vi "Select Worksheet for Logging.vi"(11 "Excel Logger.lvclass":refnum<class "Excel Logger.lvclass">) -> (0 "Canceled":bool=TRUE, 3 "Excel Logger.lvclass 2":refnum<class "Excel Logger.lvclass">)   [LabVIEW 2013, in "Excel Logger.lvclass"]
uses:
  Excel Logger.lvclass
  Excel Logger.lvclass/Excel Logger.ctl
  Excel Interface/Excel Interface.lvclass
  Data Analyser Report/Data Analyser Report.lvclass
panel:
  in  "Text":bool
  in  "Cancel":bool
  in  "OK Button":bool
  # "Please sellect now the worksheet that you \nwould like to use for saving the \n                                   \n\nWhen you are done press OK"
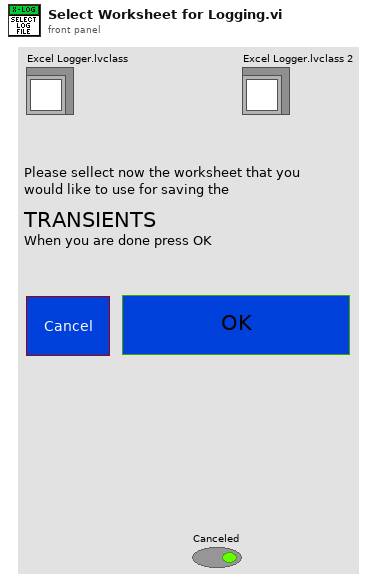
[diagram p1: front panel]
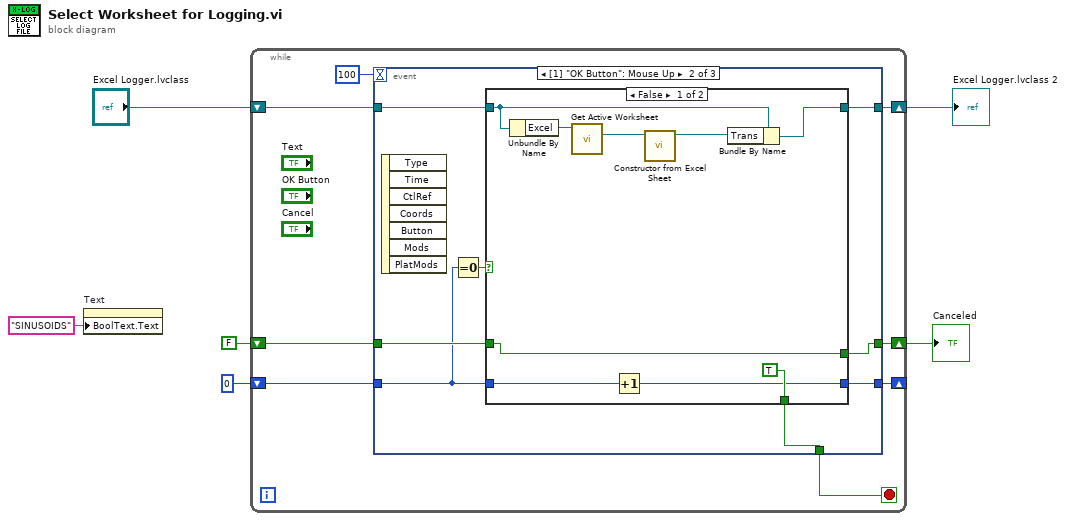
[diagram p0: block diagram]
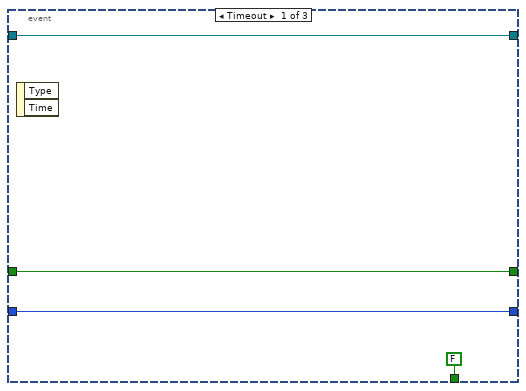
[diagram p2: hidden frame]
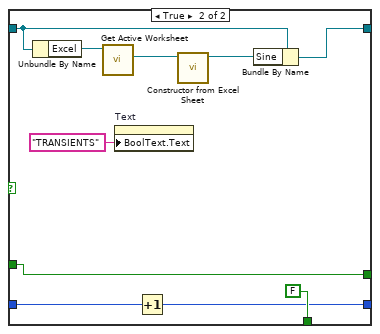
[diagram p3: hidden frame]
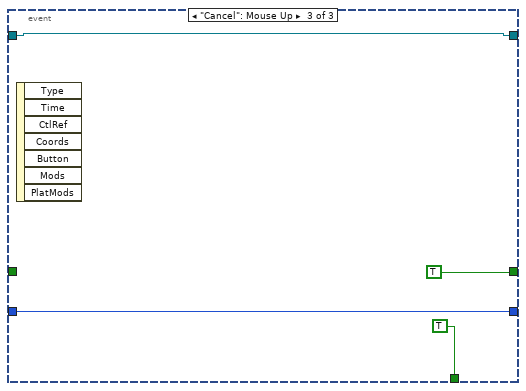
[diagram p4: hidden frame]
diagram:
  n1 = property on="Text" class="Bool"("BoolText.Text"="SINUSOIDS" ("Boolean Text.Text")) -> ()  [unwired: 2 in, 2 out]
  n2 = while {
    shift-right: [w9] -> w4
    shift-left: FALSE -> [w12]
    shift-right: [w10] -> _
    shift-left: 0 -> [w11]
    shift-right: [w7] -> w2
    shift-left: "Excel Logger.lvclass" -> [w8]
    stop <- w13 stop-if-true
    n3 = event shown="[1] \"OK Button\": Mouse Up" {
      selector: _ -> [_ _ _]
      dyn-events: _ -> [_ _ _]
      timeout: 100 -> [_ _ _]
      tunnel: [FALSE w26 TRUE] -> w13
      tunnel: w12 -> [w16 w25 _]
      tunnel: w11 -> [w17 w23 w48]
      tunnel: [w17 w22 w48] -> w10
      tunnel: [w16 w19 TRUE] -> w9
      tunnel: w8 -> [w15 w21 w46]
      tunnel: [w15 w20 w46] -> w7
      event Timeout {
        n4 = event-data() -> ()  [unwired: 1 in, 2 out]
      }
      event "OK Button": Mouse Up {
        n5 = event-data() -> ()  [unwired: 1 in, 7 out]
        n6 = Equal To 0?(x=w23) -> (x = 0?=w24:bool)
        n7 = case shown="False" w24 {
          tunnel: [TRUE FALSE] -> w26
          tunnel: w25 -> [w32 w42]
          tunnel: w23 -> [w34 w44]
          tunnel: [w33 w43] -> w22
          tunnel: w21 -> [w30 w40]
          tunnel: [w29 w39] -> w20
          tunnel: [w32 w42] -> w19
          frame False {
            n8 = Unbundle By Name(w30) -> ("Excel"=w31:refnum<class "Excel Interface.lvclass">)
            n9 = call-dynamic "Get Active Worksheet.vi"("Excel Interface in"=w31) -> ("Excel Sheet out"=w28:refnum<class "Excel Sheet.lvclass">)  [unwired: 8 in, 2 out]
            n10 = Increment(x=w34) -> (x+1=w33:i32)
            n11 = call "Constructor from Excel Sheet.vi"("Excel Sheet.lvclass"=w28) -> ("Data Analyser Report.lvclass"=w27:refnum<class "Data Analyser Report.lvclass">)  [unwired: 10 in]
            n12 = Bundle By Name(cluster=w30, "Trans"=w27) -> (w29:refnum<class "Excel Logger.lvclass">)
          }
          frame True {
            n13 = Unbundle By Name(w40) -> ("Excel"=w41:refnum<class "Excel Interface.lvclass">)
            n14 = call-dynamic "Get Active Worksheet.vi"("Excel Interface in"=w41) -> ("Excel Sheet out"=w37:refnum<class "Excel Sheet.lvclass">)  [unwired: 8 in, 2 out]
            n15 = property on="Text" class="Bool"("BoolText.Text"="TRANSIENTS" ("Boolean Text.Text")) -> ()  [unwired: 2 in, 2 out]
            n16 = Increment(x=w44) -> (x+1=w43:i32)
            n17 = call "Constructor from Excel Sheet.vi"("Excel Sheet.lvclass"=w37) -> ("Data Analyser Report.lvclass"=w36:refnum<class "Data Analyser Report.lvclass">)  [unwired: 10 in]
            n18 = Bundle By Name(cluster=w40, "Sine"=w36) -> (w39:refnum<class "Excel Logger.lvclass">)
          }
        }
      }
      event "Cancel": Mouse Up {
        n19 = event-data() -> ()  [unwired: 1 in, 7 out]
      }
    }
  }
  "Canceled" <- w4
  "Excel Logger.lvclass 2" <- w2
